vi "AutoSequences.vi"() -> ()   [LabVIEW 2014]
uses:
  TypeDefs/SRE Enum.ctl
  <vilib>/Rock Robotics/Network Tables/SD Write Boolean.vi
  <vilib>/Rock Robotics/Network Tables/SD Read Number.vi
  Support Code/Robot Global Data.vi
panel:
  out "output cluster":T1
  out "Time to hall effect":i32
  in  "Direction":dbl=1.25 format="%#_13g"
  in  "Set To":dbl=-135.0 format="%#_13g"
  in  "Angle":dbl=-155.0 format="%#_13g"
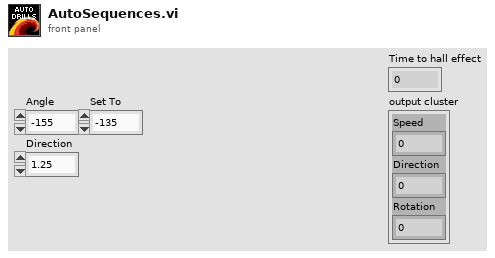
[diagram p1: front panel]
types:
  T1 = cluster{"Speed":dbl, "Direction":dbl, "Rotation":dbl}
  T2 = typedef "SRE Enum.ctl" = enum16{"Start", "Run", "End"}
  T3 = enum16{"High", "Middle", "Low", "Really Low", "Stopped"}
  T4 = cluster{"Duration(seconds)":i32, "Rotation(Angle)":dbl, "Direction":dbl}
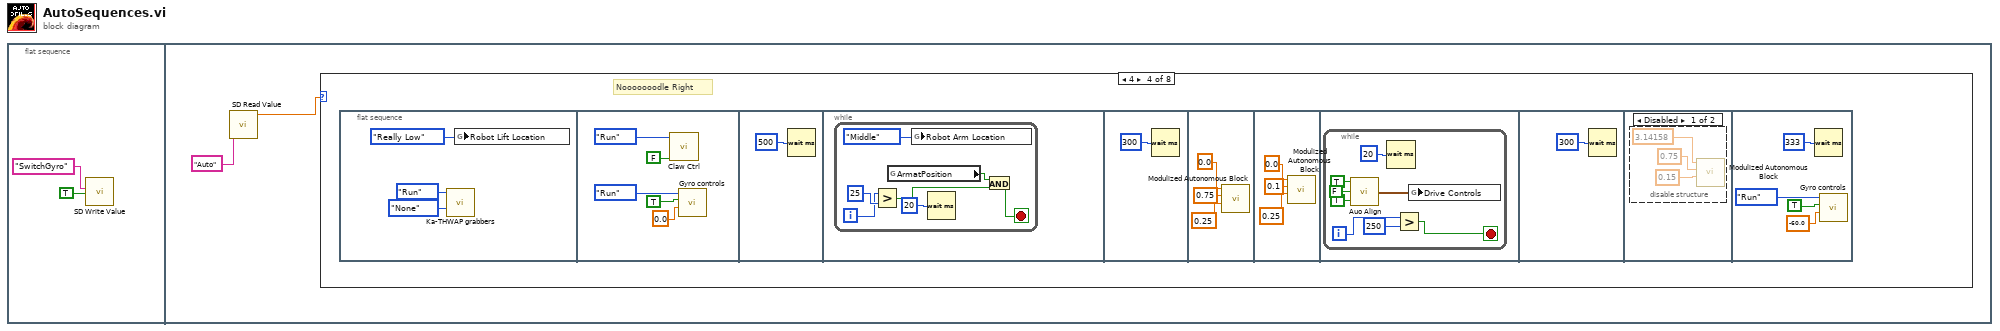
[diagram p0: block diagram]
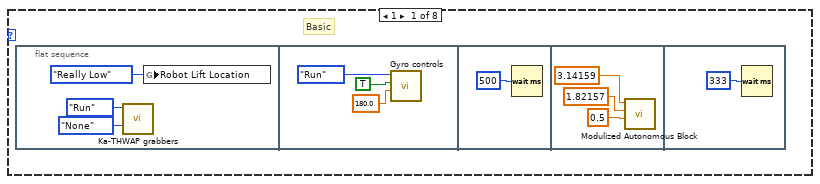
[diagram p2: hidden frame]
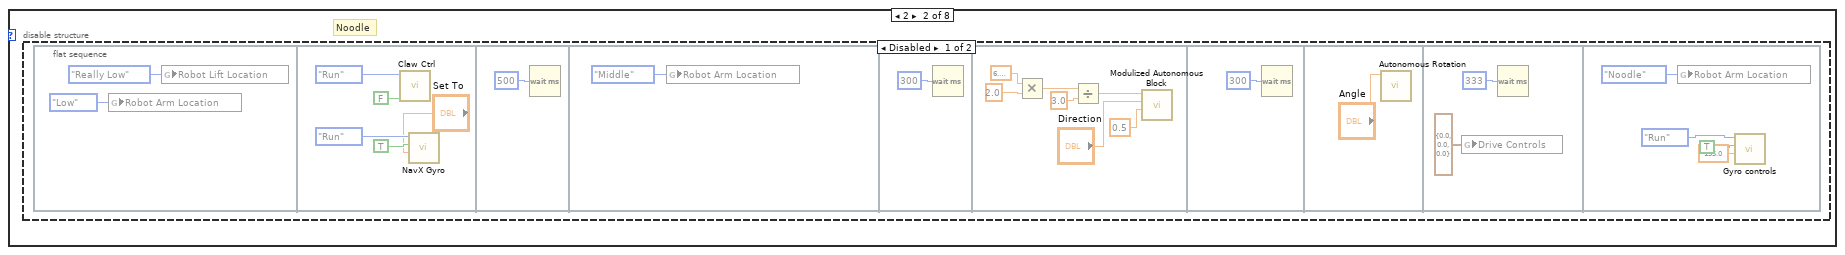
[diagram p3: hidden frame]
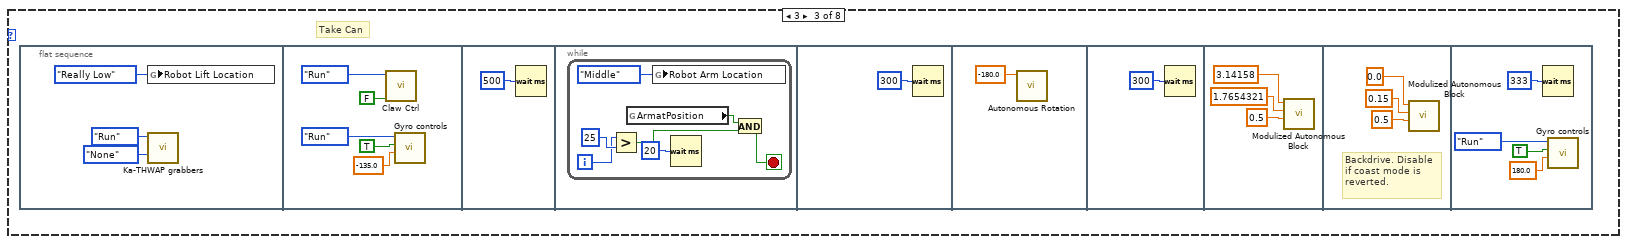
[diagram p5: hidden frame]
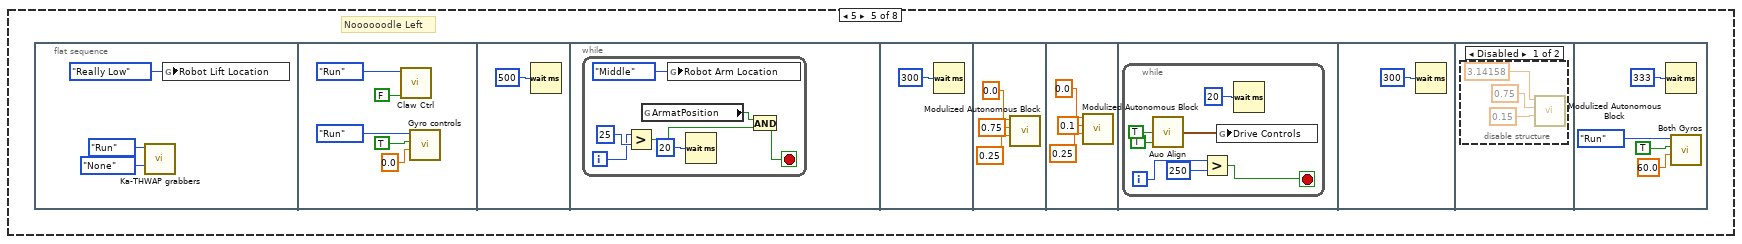
[diagram p7: hidden frame]
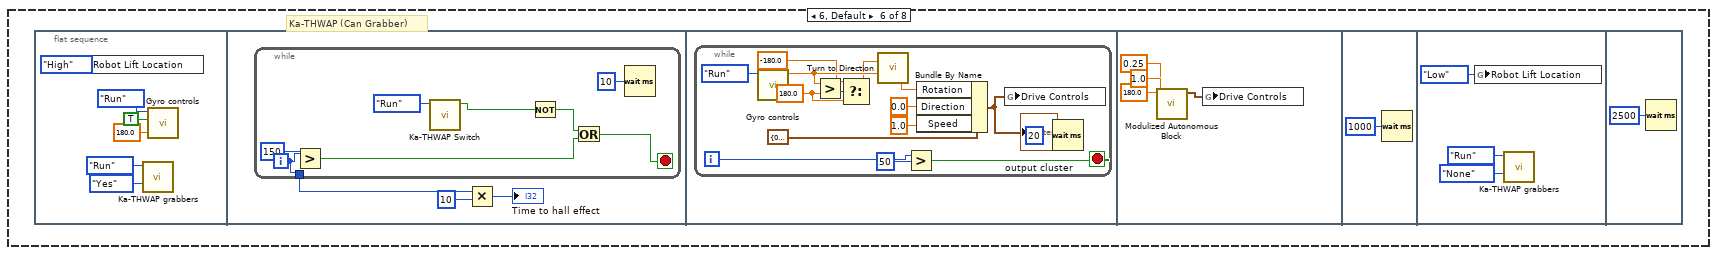
[diagram p9: hidden frame]
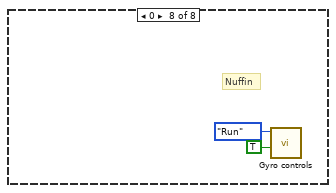
[diagram p11: hidden frame]
diagram:
  n1 = flat-sequence {
    frame #0 {
      n2 = call-poly <vilib>:"SD Write Value.vi"("Boolean"=TRUE, "Table Prefix"="SwitchGyro" ("Name")) -> ()  [unwired: 8 in, 2 out]
    }
    frame #1 {
      n3 = call-poly <vilib>:"SD Read Value.vi"("Name"="Auto") -> ("Numeric"=w4:dbl)  [unwired: 8 in, 2 out]
      n4 = case shown="4" w4 {
        frame 1 {
          # "Basic"
          n5 = flat-sequence {
            frame #0 {
              n6 = call "Ka-THWAP grabbers.vi"("Action"=enum16{"None", "Left", "Right", "Yes"}."None", "Enum"=SRE_Enum."Run") -> ()  [unwired: 10 in]
              n7 = global write "Robot Global Data.vi" "Robot Lift Location"(enum16{"High", "Middle", "Low", "Really Low"}."Really Low" ("Robot Lift Location")) -> ()
            }
            frame #1 {
              n8 = call "Gyro controls.vi"("Set To"=180.0, "Reset"=TRUE, "Enum"=SRE_Enum."Run") -> ()  [unwired: 8 in, 1 out]
            }
            frame #2 {
              n9 = Wait (ms)(milliseconds to wait=u32 500) -> ()  [unwired: 1 out]
            }
            frame #3 {
              n10 = call "Modulized Autonomous Block.vi"("Power"=0.5, "run time in seconds"=1.82157 ("Direction"), "Direction"=3.14159) -> ()  [unwired: 8 in, 1 out]
            }
            frame #4 {
              n11 = Wait (ms)(milliseconds to wait=u32 333) -> ()  [unwired: 1 out]
            }
          }
        }
        frame 2 {
          # "Noodle"
          n12 = disable-structure shown="Disabled" {
            frame Disabled {
              n13 = flat-sequence {
                frame #0 {
                  n14 = global write "Robot Global Data.vi" "Robot Arm Location"(enum16{"High", "Middle", "Low", "Noodle"}."Low" ("Robot Arm Location")) -> ()
                  n15 = global write "Robot Global Data.vi" "Robot Lift Location"(enum16{"High", "Middle", "Low", "Really Low"}."Really Low" ("Robot Lift Location")) -> ()
                }
                frame #1 {
                  n16 = call "Claw Ctrl.vi"("Open/Close"=FALSE, "Enum"=SRE_Enum."Run") -> ()  [unwired: 10 in]
                  n17 = call "NavX Gyro.vi"("Set To"="Set To", "Reset"=TRUE, "Enum"=SRE_Enum."Run") -> ()  [unwired: 6 in, 3 out]
                }
                frame #2 {
                  n18 = Wait (ms)(milliseconds to wait=u32 500) -> ()  [unwired: 1 out]
                }
                frame #3 {
                  n19 = global write "Robot Global Data.vi" "Robot Arm Location"(enum16{"High", "Middle", "Low", "Noodle"}."Middle" ("Robot Arm Location")) -> ()
                }
                frame #4 {
                  n20 = Wait (ms)(milliseconds to wait=u32 300) -> ()  [unwired: 1 out]
                }
                frame #5 {
                  n21 = Multiply(x=6.283185307179586, y=2.0) -> (x*y=w29:dbl)
                  n22 = Divide(x=w29, y=3.0) -> (x/y=w27:dbl)
                  n23 = call "Modulized Autonomous Block.vi"("Power"=0.5, "run time in seconds"="Direction", "Direction"=w27) -> ()  [unwired: 8 in, 1 out]
                }
                frame #6 {
                  n24 = Wait (ms)(milliseconds to wait=u32 300) -> ()  [unwired: 1 out]
                }
                frame #7 {
                  n25 = call "Autonomous Rotation.vi"("Angle"="Angle") -> ()  [unwired: 11 in]
                }
                frame #8 {
                  n26 = global write "Robot Global Data.vi" "Drive Controls"(T1 {"Speed"=0.0, "Direction"=0.0, "Rotation"=0.0} ("Drive Controls")) -> ()
                  n27 = Wait (ms)(milliseconds to wait=u32 333) -> ()  [unwired: 1 out]
                }
                frame #9 {
                  n28 = global write "Robot Global Data.vi" "Robot Arm Location"(enum16{"High", "Middle", "Low", "Noodle"}."Noodle" ("Robot Arm Location")) -> ()
                  n29 = call "Gyro controls.vi"("Set To"=-155.0, "Reset"=TRUE, "Enum"=SRE_Enum."Run") -> ()  [unwired: 8 in, 1 out]
                }
              }
            }
            frame Enabled {
            }
          }
        }
        frame 3 {
          # "Take Can"
          n30 = flat-sequence {
            frame #0 {
              n31 = global write "Robot Global Data.vi" "Robot Lift Location"(enum16{"High", "Middle", "Low", "Really Low"}."Really Low" ("Robot Lift Location")) -> ()
              n32 = call "Ka-THWAP grabbers.vi"("Action"=enum16{"None", "Left", "Right", "Yes"}."None", "Enum"=SRE_Enum."Run") -> ()  [unwired: 10 in]
            }
            frame #1 {
              n33 = call "Claw Ctrl.vi"("Open/Close"=FALSE, "Enum"=SRE_Enum."Run") -> ()  [unwired: 10 in]
              n34 = call "Gyro controls.vi"("Set To"=-135.0, "Reset"=TRUE, "Enum"=SRE_Enum."Run") -> ()  [unwired: 8 in, 1 out]
            }
            frame #2 {
              n35 = Wait (ms)(milliseconds to wait=u32 500) -> ()  [unwired: 1 out]
            }
            frame #3 {
              n36 = while {
                i -> [w50]
                stop <- w54 stop-if-true
                n37 = Greater?(x=w50, y=25 ("x")) -> (0:w52:bool)
                n38 = global read "Robot Global Data.vi" "ArmatPosition"() -> (w53:bool)
                n39 = global write "Robot Global Data.vi" "Robot Arm Location"(enum16{"High", "Middle", "Low", "Noodle"}."Middle" ("Robot Arm Location")) -> ()
                n40 = Wait (ms)(milliseconds to wait=u32 20) -> ()  [unwired: 1 out]
                n41 = And(x=w53, y=w52) -> (x .and. y?=w54:bool)
              }
            }
            frame #4 {
              n42 = Wait (ms)(milliseconds to wait=u32 300) -> ()  [unwired: 1 out]
            }
            frame #5 {
              n43 = call "Autonomous Rotation.vi"("Angle"=-180.0) -> ()  [unwired: 11 in]
            }
            frame #6 {
              n44 = Wait (ms)(milliseconds to wait=u32 300) -> ()  [unwired: 1 out]
            }
            frame #7 {
              n45 = call "Modulized Autonomous Block.vi"("Power"=0.5, "run time in seconds"=1.7654321 ("Direction"), "Direction"=3.14158) -> ()  [unwired: 8 in, 1 out]
            }
            frame #8 {
              # "Backdrive. Disable\nif coast mode is\nreverted."
              n46 = call "Modulized Autonomous Block.vi"("Power"=0.5, "run time in seconds"=0.15 ("Direction"), "Direction"=0.0) -> ()  [unwired: 8 in, 1 out]
            }
            frame #9 {
              n47 = Wait (ms)(milliseconds to wait=u32 333) -> ()  [unwired: 1 out]
              n48 = call "Gyro controls.vi"("Set To"=180.0, "Reset"=TRUE, "Enum"=SRE_Enum."Run") -> ()  [unwired: 8 in, 1 out]
            }
          }
        }
        frame 4 {
          # "Nooooooodle Right"
          n49 = flat-sequence {
            frame #0 {
              n50 = call "Ka-THWAP grabbers.vi"("Action"=enum16{"None", "Left", "Right", "Yes"}."None", "Enum"=SRE_Enum."Run") -> ()  [unwired: 10 in]
              n51 = global write "Robot Global Data.vi" "Robot Lift Location"(enum16{"High", "Middle", "Low", "Really Low"}."Really Low" ("Robot Lift Location")) -> ()
            }
            frame #1 {
              n52 = call "Claw Ctrl.vi"("Open/Close"=FALSE, "Enum"=SRE_Enum."Run") -> ()  [unwired: 10 in]
              n53 = call "Gyro controls.vi"("Set To"=0.0, "Reset"=TRUE, "Enum"=SRE_Enum."Run") -> ()  [unwired: 8 in, 1 out]
            }
            frame #2 {
              n54 = Wait (ms)(milliseconds to wait=u32 500) -> ()  [unwired: 1 out]
            }
            frame #3 {
              n55 = while {
                i -> [w79]
                stop <- w83 stop-if-true
                n56 = Greater?(x=w79, y=25 ("x")) -> (0:w81:bool)
                n57 = global read "Robot Global Data.vi" "ArmatPosition"() -> (w82:bool)
                n58 = global write "Robot Global Data.vi" "Robot Arm Location"(enum16{"High", "Middle", "Low", "Noodle"}."Middle" ("Robot Arm Location")) -> ()
                n59 = Wait (ms)(milliseconds to wait=u32 20) -> ()  [unwired: 1 out]
                n60 = And(x=w82, y=w81) -> (x .and. y?=w83:bool)
              }
            }
            frame #4 {
              n61 = Wait (ms)(milliseconds to wait=u32 300) -> ()  [unwired: 1 out]
            }
            frame #5 {
              n62 = call "Modulized Autonomous Block.vi"("Power"=0.25, "run time in seconds"=0.75, "Direction"=0.0) -> ()  [unwired: 8 in, 1 out]
            }
            frame #6 {
              n63 = call "Modulized Autonomous Block.vi"("Power"=0.25, "run time in seconds"=0.1, "Direction"=0.0) -> ()  [unwired: 8 in, 1 out]
            }
            frame #7 {
              n64 = while {
                i -> [w98]
                stop <- w96 stop-if-true
                n65 = call "Auo Align.vi"("Noodle?"=TRUE, "RotateRight"=FALSE, "RotateLeft"=TRUE) -> ("output cluster"=w99:T1)
                n66 = Wait (ms)(milliseconds to wait=u32 20) -> ()  [unwired: 1 out]
                n67 = Greater?(x=w98, y=250) -> (0:w96:bool)
                n68 = global write "Robot Global Data.vi" "Drive Controls"(w99) -> ()
              }
            }
            frame #8 {
              n69 = Wait (ms)(milliseconds to wait=u32 300) -> ()  [unwired: 1 out]
            }
            frame #9 {
              n70 = disable-structure shown="Disabled" {
                frame Disabled {
                  n71 = call "Modulized Autonomous Block.vi"("Power"=0.15, "run time in seconds"=0.75 ("Direction"), "Direction"=3.14158) -> ()  [unwired: 8 in, 1 out]
                }
                frame Enabled {
                }
              }
            }
            frame #10 {
              n72 = Wait (ms)(milliseconds to wait=u32 333) -> ()  [unwired: 1 out]
              n73 = call "Gyro controls.vi"("Set To"=-60.0, "Reset"=TRUE, "Enum"=SRE_Enum."Run") -> ()  [unwired: 8 in, 1 out]
            }
          }
        }
        frame 5 {
          # "Noooooodle Left"
          n74 = flat-sequence {
            frame #0 {
              n75 = call "Ka-THWAP grabbers.vi"("Action"=enum16{"None", "Left", "Right", "Yes"}."None", "Enum"=SRE_Enum."Run") -> ()  [unwired: 10 in]
              n76 = global write "Robot Global Data.vi" "Robot Lift Location"(enum16{"High", "Middle", "Low", "Really Low"}."Really Low" ("Robot Lift Location")) -> ()
            }
            frame #1 {
              n77 = call "Claw Ctrl.vi"("Open/Close"=FALSE, "Enum"=SRE_Enum."Run") -> ()  [unwired: 10 in]
              n78 = call "Gyro controls.vi"("Set To"=0.0, "Reset"=TRUE, "Enum"=SRE_Enum."Run") -> ()  [unwired: 8 in, 1 out]
            }
            frame #2 {
              n79 = Wait (ms)(milliseconds to wait=u32 500) -> ()  [unwired: 1 out]
            }
            frame #3 {
              n80 = while {
                i -> [w118]
                stop <- w122 stop-if-true
                n81 = Greater?(x=w118, y=25 ("x")) -> (0:w120:bool)
                n82 = global read "Robot Global Data.vi" "ArmatPosition"() -> (w121:bool)
                n83 = global write "Robot Global Data.vi" "Robot Arm Location"(enum16{"High", "Middle", "Low", "Noodle"}."Middle" ("Robot Arm Location")) -> ()
                n84 = Wait (ms)(milliseconds to wait=u32 20) -> ()  [unwired: 1 out]
                n85 = And(x=w121, y=w120) -> (x .and. y?=w122:bool)
              }
            }
            frame #4 {
              n86 = Wait (ms)(milliseconds to wait=u32 300) -> ()  [unwired: 1 out]
            }
            frame #5 {
              n87 = call "Modulized Autonomous Block.vi"("Power"=0.25, "run time in seconds"=0.75, "Direction"=0.0) -> ()  [unwired: 8 in, 1 out]
            }
            frame #6 {
              n88 = call "Modulized Autonomous Block.vi"("Power"=0.25, "run time in seconds"=0.1, "Direction"=0.0) -> ()  [unwired: 8 in, 1 out]
            }
            frame #7 {
              n89 = while {
                i -> [w136]
                stop <- w134 stop-if-true
                n90 = call "Auo Align.vi"("Noodle?"=TRUE, "RotateRight"=TRUE) -> ("output cluster"=w137:T1)  [unwired: 1 in]
                n91 = Greater?(x=w136, y=250) -> (0:w134:bool)
                n92 = global write "Robot Global Data.vi" "Drive Controls"(w137) -> ()
                n93 = Wait (ms)(milliseconds to wait=u32 20) -> ()  [unwired: 1 out]
              }
            }
            frame #8 {
              n94 = Wait (ms)(milliseconds to wait=u32 300) -> ()  [unwired: 1 out]
            }
            frame #9 {
              n95 = disable-structure shown="Disabled" {
                frame Disabled {
                  n96 = call "Modulized Autonomous Block.vi"("Power"=0.15, "run time in seconds"=0.75 ("Direction"), "Direction"=3.14158) -> ()  [unwired: 8 in, 1 out]
                }
                frame Enabled {
                }
              }
            }
            frame #10 {
              n97 = Wait (ms)(milliseconds to wait=u32 333) -> ()  [unwired: 1 out]
              n98 = call "Both Gyros.vi"("Set To"=60.0, "Reset"=TRUE, "Enum"=SRE_Enum."Run") -> ()  [unwired: 8 in, 1 out]
            }
          }
        }
        frame 6, Default {
          # "Ka-THWAP (Can Grabber)"
          n99 = flat-sequence {
            frame #0 {
              n100 = global write "Robot Global Data.vi" "Robot Lift Location"(T3."High" ("Robot Lift Location")) -> ()
              n101 = call "Ka-THWAP grabbers.vi"("Action"=enum16{"None", "Left", "Right", "Yes"}."Yes", "Enum"=SRE_Enum."Run") -> ()  [unwired: 10 in]
              n102 = call "Gyro controls.vi"("Set To"=180.0, "Reset"=TRUE, "Enum"=SRE_Enum."Run") -> ()  [unwired: 8 in, 1 out]
            }
            frame #1 {
              n103 = while {
                tunnel: [w156] -> w155
                i -> [w156]
                stop <- w157 stop-if-true
                n104 = Greater?(x=w156, y=150) -> (0:w158:bool)
                n105 = call "Ka-THWAP Switch.vi"("Run Mode"=SRE_Enum."Run") -> ("Value"=w160:bool)  [unwired: 10 in]
                n106 = Not(x=w160) -> (.not. x?=w159:bool)
                n107 = Or(x=w159, y=w158) -> (x .or. y?=w157:bool)
                n108 = Wait (ms)(milliseconds to wait=u32 10) -> ()  [unwired: 1 out]
              }
              n109 = Multiply(x=w155, y=10) -> (x*y=→"Time to hall effect":i32)
            }
            frame #2 {
              n110 = while {
                i -> [w172]
                stop <- w170 stop-if-true
                w165 = 180.0 ("y")
                n111 = call "Gyro controls.vi"("Enum"=SRE_Enum."Run") -> ("Angle"=w168:dbl)  [unwired: 10 in]
                n112 = Greater?(x=w168, y=w165) -> (0:w166:bool)
                n113 = Select(t=-180.0 ("Set"), s=w166, f=w165) -> (s? t:f=w167:dbl)
                n114 = call "Turn to Direction.vi"("Gyroscope"=w168, "Set"=w167) -> ("Rotation Speed"=w175:dbl)
                n115 = Greater?(x=w172, y=50) -> (0:w170:bool)
                n116 = Bundle By Name(cluster=T1 {"Speed"=0.0, "Direction"=0.0, "Rotation"=0.0} ("Drive Controls"), "Rotation"=w175, "Direction"=0.0, "Speed"=1.0) -> (w174:T1)
                "output cluster" <- w174
                n117 = global write "Robot Global Data.vi" "Drive Controls"(w174) -> ()
                n118 = Wait (ms)(milliseconds to wait=u32 20) -> ()  [unwired: 1 out]
              }
            }
            frame #3 {
              n119 = call "Modulized Autonomous Block.vi"("Power"=1.0, "run time in seconds"=0.25, "Direction"=180.0) -> ("Output"=w182:T4)  [unwired: 8 in]
              n120 = global write "Robot Global Data.vi" "Drive Controls"(w182) -> ()
            }
            frame #4 {
              n121 = Wait (ms)(milliseconds to wait=u32 1000) -> ()  [unwired: 1 out]
            }
            frame #5 {
              n122 = global write "Robot Global Data.vi" "Robot Lift Location"(T3."Low" ("Robot Lift Location")) -> ()
              n123 = call "Ka-THWAP grabbers.vi"("Action"=enum16{"None", "Left", "Right", "Yes"}."None", "Enum"=SRE_Enum."Run") -> ()  [unwired: 10 in]
            }
            frame #6 {
              n124 = Wait (ms)(milliseconds to wait=u32 2500) -> ()  [unwired: 1 out]
            }
          }
        }
        frame 7 {
        }
        frame 0 {
          # "Nuffin"
          n125 = call "Gyro controls.vi"("Reset"=TRUE, "Enum"=SRE_Enum."Run") -> ()  [unwired: 9 in, 1 out]
        }
      }
    }
  }
